vi "RichToFlatni_measurementlink_pinmap_v1_QueryResourceAccessInformationResponse.vi"(5 "OutputClusterType":T1, 11 "InputCluster":T4) -> (3 "OutputCluster":T1)   [LabVIEW 2020, in "MeasurementLink Pin Map Client.lvlib"]
uses:
  MeasurementLink Pin Map Client.lvlib
  ni_measurementlink_pinmap_v1_QueryResourceAccessInformationResponse.ctl
  ni_measurementlink_pinmap_v1_ResourceAccessInformation.ctl
  ni_measurementlink_pinmap_v1_ChannelMapping.ctl
  ni_measurementlink_pinmap_v1_QueryResourceAccessInformationResponse_Flat.ctl
  ni_measurementlink_pinmap_v1_ResourceAccessInformation_Flat.ctl
  ni_measurementlink_pinmap_v1_ChannelMapping_Flat.ctl
  RichToFlatni_measurementlink_pinmap_v1_ChannelMapping.vi
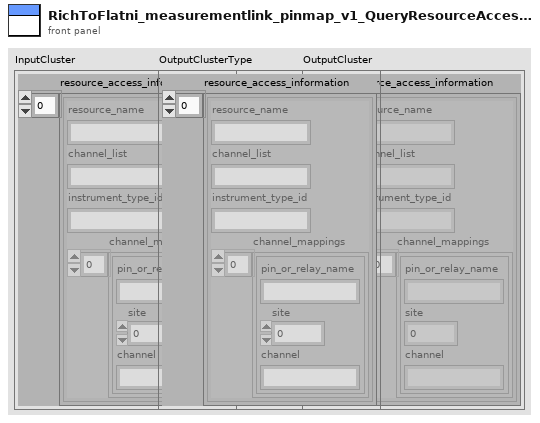
[diagram p1: front panel]
types:
  T1 = typedef "MeasurementLink Pin Map Client.lvlib/ni_measurementlink_pinmap_v1_QueryResourceAccessInformationResponse_Flat.ctl" = cluster{"resource_access_information":T2[]}
  T2 = typedef "MeasurementLink Pin Map Client.lvlib/ni_measurementlink_pinmap_v1_ResourceAccessInformation_Flat.ctl" = cluster{"resource_name":string, "channel_list":string, "instrument_type_id":string, "channel_mappings":T3[]}
  T3 = typedef "MeasurementLink Pin Map Client.lvlib/ni_measurementlink_pinmap_v1_ChannelMapping_Flat.ctl" = cluster{"pin_or_relay_name":string, "site":i32, "channel":string}
  T4 = typedef "MeasurementLink Pin Map Client.lvlib/ni_measurementlink_pinmap_v1_QueryResourceAccessInformationResponse.ctl" = cluster{"resource_access_information":T5[]}
  T5 = typedef "MeasurementLink Pin Map Client.lvlib/ni_measurementlink_pinmap_v1_ResourceAccessInformation.ctl" = cluster{"resource_name":string, "channel_list":string, "instrument_type_id":string, "channel_mappings":T6[]}
  T6 = typedef "MeasurementLink Pin Map Client.lvlib/ni_measurementlink_pinmap_v1_ChannelMapping.ctl" = cluster{"pin_or_relay_name":string, "site":i32, "channel":string}
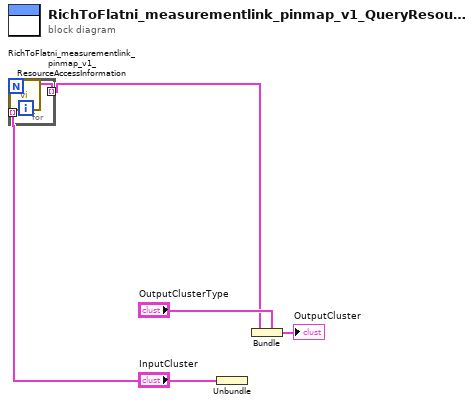
[diagram p0: block diagram]
diagram:
  n1 = Unbundle "Unbundle"("InputCluster") -> ("resource_access_information"=w2:T5[])
  n2 = for {
    tunnel: w2 -> [w7] mode=indexing
    tunnel: [w6] -> w1 mode=indexing
    n3 = call "RichToFlatni_measurementlink_pinmap_v1_ResourceAccessInformation.vi"("InputCluster"=w7) -> ("OutputCluster"=w6:T2)  [unwired: 10 in]
  }
  n4 = Bundle "Bundle"(cluster="OutputClusterType", "resource_access_information"=w1) -> (→"OutputCluster":T1)
